vi "StopDrive.vi"(8 "error in (no error)":errorcluster, 11 "Stand in":refnum<class "Stand.lvclass">) -> (0 "error out":errorcluster, 3 "Stand out":refnum<class "Stand.lvclass">)   [LabVIEW 2019, in "Stand.lvclass"]
uses:
  Stand.lvclass
  Stand.lvclass/Stand.ctl
  dY_dX_Calculator/delayValue.lvclass/delayValue.ctl
  FPGA/TypeDef/AI index.ctl
  AI_class/AI.lvclass/AI.ctl
  AnalogComparator_class/AnalogComparator.lvclass/AnalogComparator.ctl
  21761a90-0765-4886-8535-fe51b9291983.vi
  <vilib>/Utility/error.llb/Clear Errors.vi
  AnalogComparator_class/GetStatus.vi
  dY_dX_Calculator/delayValue.lvclass
  AI_class/AI.lvclass
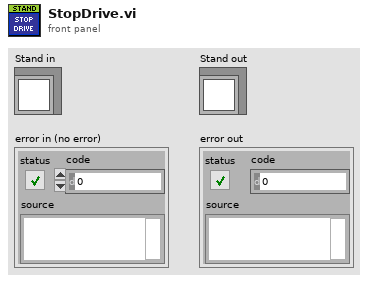
[diagram p1: front panel]
types:
  T1 = typedef "AI index.ctl" = u8
  T2 = typedef "AI_Data.ctl" = cluster{"Stat Data":T3, "OutOfRangeMax":bool, "OutOfRangeMin":bool, "HIHI":bool, "HI":bool, "LO":bool, "LOLO":bool}
  T3 = typedef "AI Statistics Data.ctl" = cluster{"raw mean":dbl, "scl mean":dbl, "raw mean 1Hz":dbl, "scl mean 1Hz":dbl}
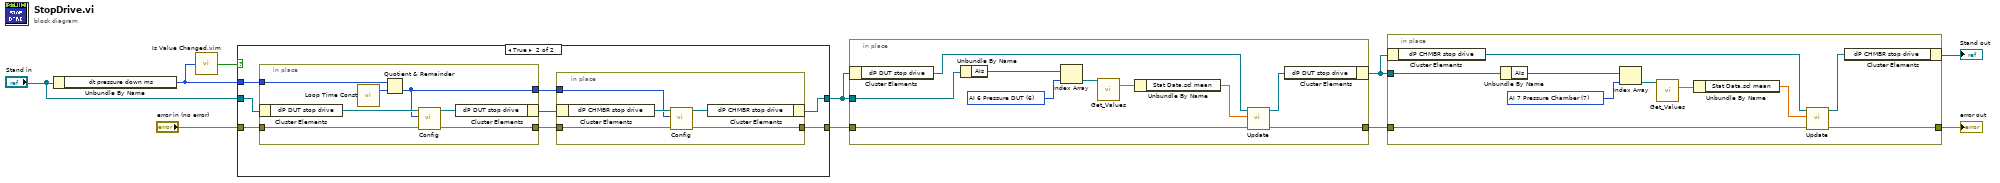
[diagram p0: block diagram]
diagram:
  n1 = Unbundle By Name("Stand in") -> ("dt pressure down ms"=w4:i32)
  n2 = call "Is Value Changed.vim"("value"=w4) -> ("changed or first call?"=w3:bool)
  n3 = case shown="True" w3 {
    tunnel: "error in (no error)" -> [w11 w20]
    tunnel: "Stand in" -> [w12 w19]
    tunnel: w4 -> [_ w18]
    tunnel: [w12 w16] -> w2
    tunnel: [w11 w14] -> w1
    frame False {
    }
    frame True {
      n4 = in-place {
        in-place-border: w20 -> [w29]
        in-place-border: [w28] -> w15
        in-place-border: w18 -> [w27]
        in-place-border: [w26] -> w13
        n5 = in-place-cluster #1(w19) -> ("dP DUT stop drive"=w32:refnum<class "delayValue.lvclass">)
        n6 = call "Loop Time Const.vi"() -> ("loop time ms"=w30:i64)  [unwired: 3 in]
        n7 = Quotient & Remainder(x=w27, y=w30) -> (floor(x/y)=w26:i64)  [unwired: 1 out]
        n8 = call "Config.vi"("error in (no error)"=w29, "size (10)"=w26, "dY_dX_Calculator in"=w32) -> ("error out"=w28:errorcluster, "dY_dX_Calculator out"=w31:refnum<class "delayValue.lvclass">)  [unwired: 7 in]
        n9 = in-place-cluster #1("dP DUT stop drive"=w31) -> (w17:refnum<class "Stand.lvclass">)
      }
      n10 = in-place {
        in-place-border: w15 -> [w23]
        in-place-border: [w22] -> w14
        in-place-border: w13 -> [w21]
        n11 = in-place-cluster #2(w17) -> ("dP CHMBR stop drive"=w25:refnum<class "delayValue.lvclass">)
        n12 = call "Config.vi"("error in (no error)"=w23, "size (10)"=w21, "dY_dX_Calculator in"=w25) -> ("error out"=w22:errorcluster, "dY_dX_Calculator out"=w24:refnum<class "delayValue.lvclass">)  [unwired: 7 in]
        n13 = in-place-cluster #2("dP CHMBR stop drive"=w24) -> (w16:refnum<class "Stand.lvclass">)
      }
    }
  }
  n14 = in-place {
    in-place-border: w1 -> [w41]
    in-place-border: [w38] -> w8
    in-place-border: w2 -> [w34]
    w35 = T1 6 items=["AI 0 Cooling Station Level", "AI 1 Cooling Station Temp", "AI 2 Oil Supply Level", "AI 3 Oil Supply Temp", "AI 4 ", "AI 5 Pressure Haskel", "AI 6 Pressure DUT", "AI 7 Pressure Chamber", "AI 8 Pressure Air inlet", "AI 9 Pressure Air outlet", "AI 10 Pressure Messure Line"] ("AI index")
    n15 = in-place-cluster #3(w2) -> ("dP DUT stop drive"=w42:refnum<class "delayValue.lvclass">)
    n16 = Unbundle By Name(w34) -> ("AIs"=w36:refnum<class "AI.lvclass">[])
    n17 = Index Array(array=w36, index=w35) -> (element=w33:refnum<class "AI.lvclass">)
    n18 = call "Get_Values.vi"("reference in"=w33) -> ("Data"=w40:T2)  [unwired: 14 in]
    n19 = Unbundle By Name(w40) -> ("Stat Data.scl mean"=w39:dbl)
    n20 = call "Update.vi"("error in (no error)"=w41, "Value"=w39, "dY_dX_Calculator in"=w42) -> ("error out"=w38:errorcluster, "dY_dX_Calculator out"=w37:refnum<class "delayValue.lvclass">)  [unwired: 7 in]
    n21 = in-place-cluster #3("dP DUT stop drive"=w37) -> (w7:refnum<class "Stand.lvclass">)
  }
  n22 = in-place {
    in-place-border: w8 -> [w51]
    in-place-border: [w50] -> w10
    in-place-border: w7 -> [w44]
    w45 = T1 7 items=["AI 0 Cooling Station Level", "AI 1 Cooling Station Temp", "AI 2 Oil Supply Level", "AI 3 Oil Supply Temp", "AI 4 ", "AI 5 Pressure Haskel", "AI 6 Pressure DUT", "AI 7 Pressure Chamber", "AI 8 Pressure Air inlet", "AI 9 Pressure Air outlet", "AI 10 Pressure Messure Line"] ("AI index")
    n23 = in-place-cluster #4(w7) -> ("dP CHMBR stop drive"=w52:refnum<class "delayValue.lvclass">)
    n24 = Unbundle By Name(w44) -> ("AIs"=w46:refnum<class "AI.lvclass">[])
    n25 = Index Array(array=w46, index=w45) -> (element=w43:refnum<class "AI.lvclass">)
    n26 = call "Get_Values.vi"("reference in"=w43) -> ("Data"=w49:T2)  [unwired: 14 in]
    n27 = Unbundle By Name(w49) -> ("Stat Data.scl mean"=w48:dbl)
    n28 = call "Update.vi"("error in (no error)"=w51, "Value"=w48, "dY_dX_Calculator in"=w52) -> ("error out"=w50:errorcluster, "dY_dX_Calculator out"=w47:refnum<class "delayValue.lvclass">)  [unwired: 7 in]
    n29 = in-place-cluster #4("dP CHMBR stop drive"=w47) -> (→"Stand out":refnum<class "Stand.lvclass">)
  }
  "error out" <- w10
